vi "Periodic Tasks.vi"(8 "error in":errorcluster) -> ()   [LabVIEW 2016]
doc: "This VI runs in parallel to other tasks. It can contain as many user-defined periodic loops as you need. These can carry out PID or other sorts of timed response."
uses:
  <vilib>/Rock Robotics/SystemInterfaces/AI/FPGA_AIChannel.ctl
  <vilib>/Rock Robotics/WPI/Accelerometer/WPI_AccelerometerRange.ctl
  <vilib>/Rock Robotics/WPI/Utilities/WPI_GetSetVariantRefNum.vi
  <vilib>/Rock Robotics/WPI/Accelerometer/InternalAccelerometer/WPI_AccelerometerInternalOpen.vi
  <vilib>/Rock Robotics/WPI/Ultrasonic/WPI_SonarMB1010AnalogOpen.vi
  <vilib>/Rock Robotics/WPI/Ultrasonic/WPI_SonarMB1010AnalogRefNum Registry Set.vi
  <vilib>/Rock Robotics/WPI/Ultrasonic/WPI_SonarMB1010AnalogGetRange.vi
  <vilib>/Rock Robotics/Network Tables/NT Write Number.vi
  <vilib>/Rock Robotics/WPI/Ultrasonic/WPI_SonarMB1010AnalogClose.vi
  <vilib>/Rock Robotics/Network Tables/NT Read Boolean.vi
  <vilib>/Rock Robotics/Network Tables/NT Write Boolean.vi
panel:
  in  "Scaling Factor":dbl=0.025
  in  "Average Bits":u8=3 max=15
  out "distance":dbl(slide)=125.0 scale=0.0..250.0 scale format="%3d"
  out "error out":errorcluster
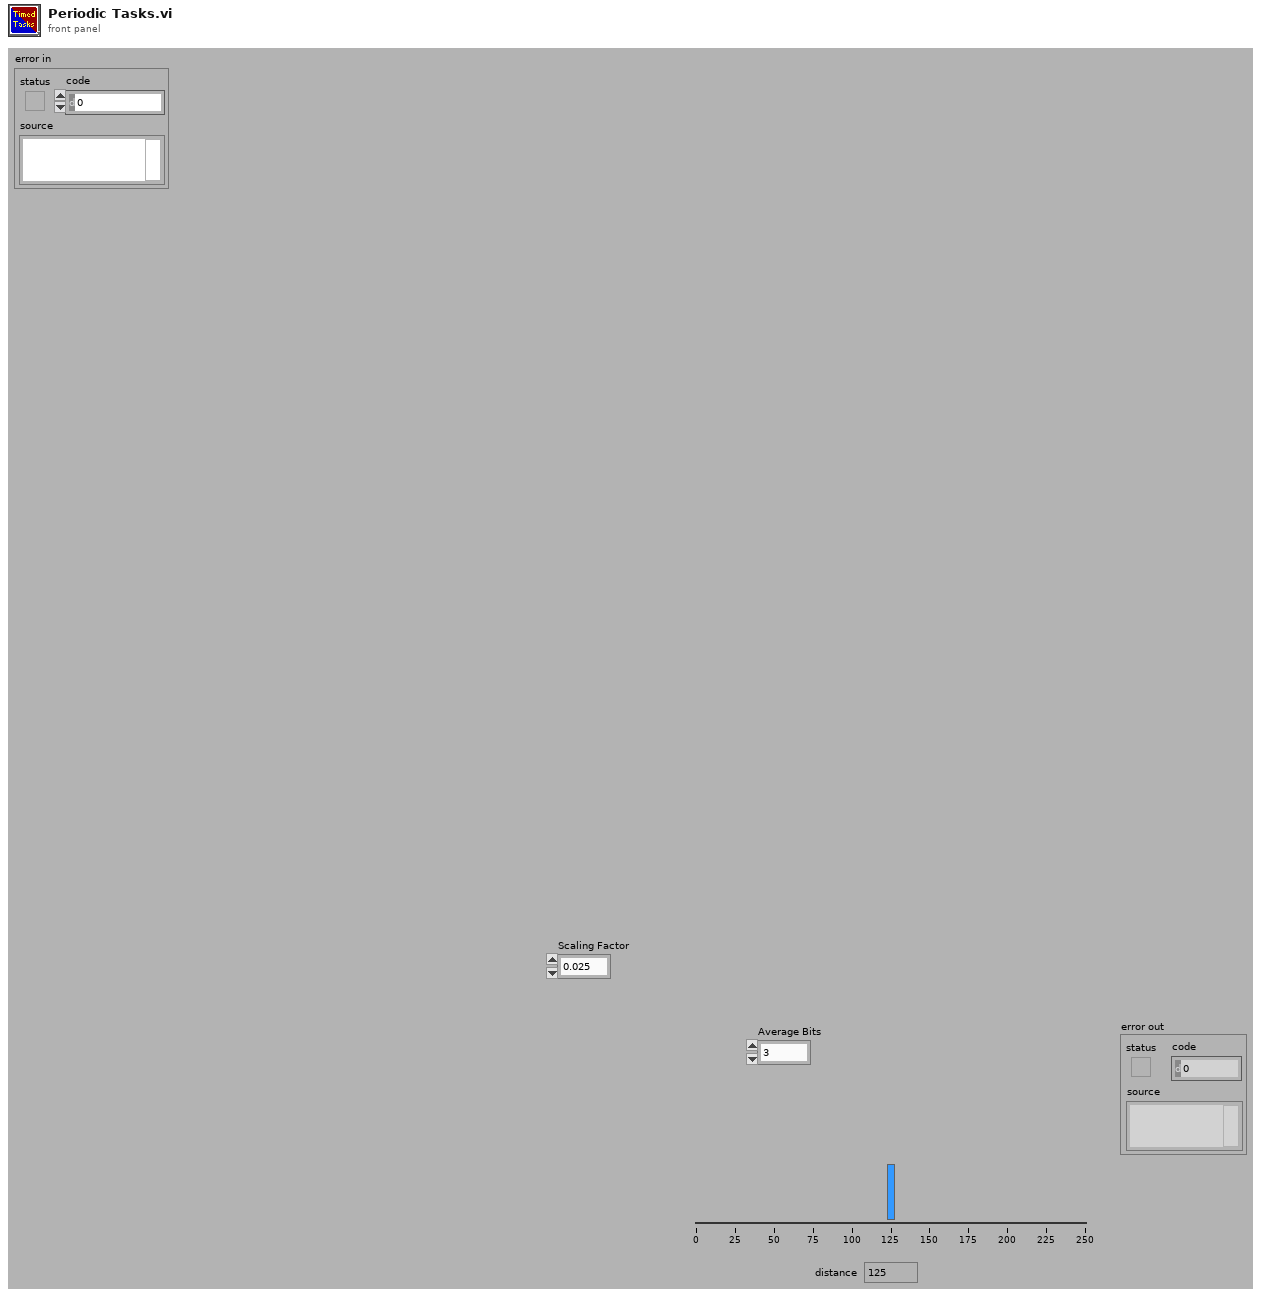
[diagram p1: front panel]
types:
  T1 = typedef "WPI_AccelerometerRange.ctl" = enum16{"+/- 2 g", "+/- 4 g", "+/- 8 g"}
  T2 = typedef "FPGA_AIChannel.ctl" = enum8{"AI 0", "AI 1", "AI 2", "AI 3", "AI MXP 0", "AI MXP 1", "AI MXP 2", "AI MXP 3", "Invalid"}
  T3 = typedef "WPI_RobotDriveDevRef.ctl" = cluster{"DevStatus":errorcluster, "Motors[]":T4[], "Square Inputs":bool, "Max Output":dbl}
  T4 = typedef "WPI_MotorControlDeviceRef.ctl" = cluster{"DeviceStatus":errorcluster, "Type":T5, "PWM":cluster{"PWM Channel":T6, "DeadBand":T7}, "CAN":cluster{"Device Number":u8, "SetOutput VI Ref":variant, "GetOutput VI Ref":variant, "Enable VI Ref":variant, "Disable VI Ref":variant, "Data":variant}, "Invert":bool}
  T5 = typedef "WPI_MotorControlType.ctl" = enum16{"PWM", "CAN"}
  T6 = typedef "FPGA_DIOPWMChannel.ctl" = enum8{"PWM 0", "PWM 1", "PWM 2", "PWM 3", "PWM 4", "PWM 5", "PWM 6", "PWM 7", "PWM 8", "PWM 9", "PWM MXP 0", "PWM MXP 1", "PWM MXP 2", "PWM MXP 3", "PWM MXP 4", "PWM MXP 5", "PWM MXP 6", "PWM MXP 7", "PWM MXP 8", "PWM MXP 9", "Invalid"}
  T7 = typedef "WPI_PWMDeadband.ctl" = cluster{"Name":string, "maxPositivePwm":i32, "minPositivePwm":i32, "centerPwm":i32, "maxNegativePwm":i32, "minNegativePwm":i32, "angularRange":u16}
  T8 = typedef "WPI_AccelerometerDevRef.ctl" = cluster{"DevStatus":errorcluster, "Scaling":T9, "Analog Channels":T10, "I2C Bus":T11, "SPI Bus":T12, "Accel Range":T13, "ADXL Axes":T14, "Handle":i32, "Device Address":u8, "Accel Type":enum16{"Analog", "ADXL345 I2C", "ADXL345 SPI", "Internal", "ADXL362 SPI"}}
  T9 = typedef "WPI_AccelerometerScaling.ctl" = cluster{"Gain (VoltsPerG)":dbl, "Center Voltage":dbl}
  T10 = typedef "WPI_AccelerometerAnalogChannels.ctl" = cluster{"X-Axis":T2, "Y-Axis":T2, "Z-Axis":T2}
  T11 = typedef "i2c_bus.ctl" = enum16{"I2C On-Board", "I2C MXP", "Invalid"}
  T12 = typedef "spi_bus.ctl" = enum16{"SPI On-Board, CS0", "SPI On-Board, CS1", "SPI On-Board, CS2", "SPI On-Board, CS3", "SPI MXP", "Invalid"}
  T13 = typedef "ADXL345 Range.ctl" = u8
  T14 = typedef "WPI_AccelerometerADXL345 Axes.ctl" = cluster{"X-Axis":bool, "Y-Axis":bool, "Z-Axis":bool}
  T15 = typedef "WPI_JoystickDevRef.ctl" = cluster{"Device":T16}
  T16 = typedef "WPI_JoystickDeviceEnum.ctl" = enum16{"USB 0", "USB 1", "USB 2", "USB 3", "USB 4", "USB 5"}
  T17 = typedef "WPI_GyroDevRef.ctl" = cluster{"DevStatus":errorcluster, "Analog Channel":T2, "Offset":dbl, "Gain (VoltsPerDegree/Second)":dbl, "Gyro Type":enum16{"Analog", "XRS450"}, "Handle":i32, "SPI Bus":T12, "Device Found":bool, "Sample Rate":dbl, "Calibrate On Open":bool}
  T18 = cluster{"JoystickDevRef":T15, "RobotDriveDevRef":T3}
  T19 = cluster{"X-Axis":dbl, "Y-Axis":dbl, "Z-Axis":dbl}
  T20 = typedef "WPI_SonarMB1010AnalogDeviceRef.ctl" = cluster{"AIDeviceRef":T21, "Scaling factor (V/in)":dbl, "Average Bits":u8}
  T21 = typedef "WPI_AnalogChannelDevRef.ctl" = cluster{"DevStatus":errorcluster, "Analog Channel":T2}
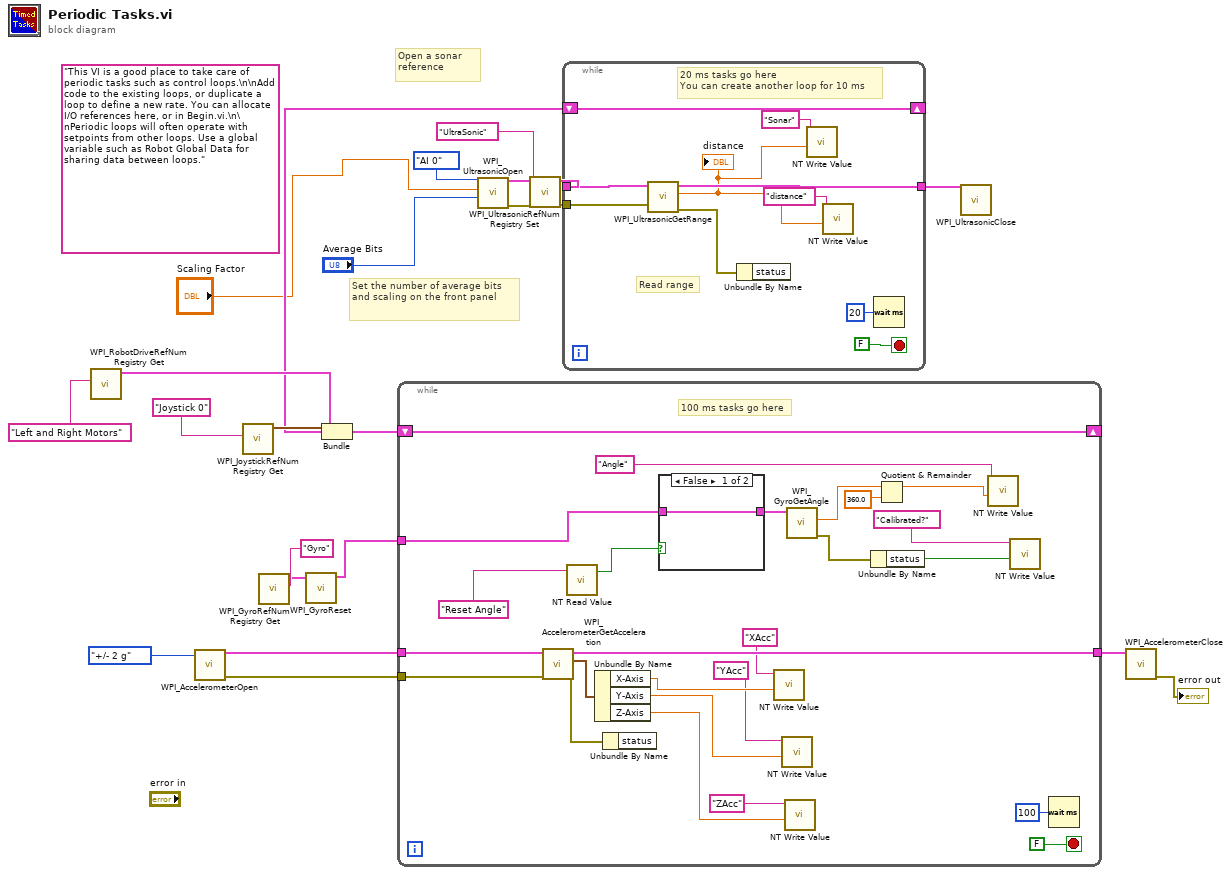
[diagram p0: block diagram]
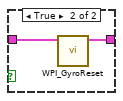
[diagram p2: hidden frame]
diagram:
  (unwired) "This VI is a good place to take care of periodic tasks such as control loops.\n\nAdd code to the existing loops, or duplicate a loop to define a new rate. You can allocate I/O references here, or in Begin.vi.\n\nPeriodic loops will often operate with setpoints from other loops. Use a global variable such as Robot Global Data for sharing data between loops."
  # "Set the number of average bits and scaling on the front panel"
  # "Open a sonar reference"
  n1 = call <vilib>:"WPI_RobotDriveRefNum Registry Get.vi"("refnum name"="Left and Right Motors") -> ("RobotDriveDevRef"=w19:T3)  [unwired: 1 in, 9 out]
  n2 = call-poly <vilib>:"WPI_AccelerometerOpen.vi"("Accel Range"=WPI_AccelerometerRange."+/- 2 g") -> ("error out"=w16:errorcluster, "AccelerometerDevRef"=w17:T8)  [unwired: 9 in]
  n3 = call <vilib>:"WPI_JoystickRefNum Registry Get.vi"("refnum name"="Joystick 0") -> ("JoystickDevRef"=w20:T15)  [unwired: 1 in, 9 out]
  n4 = call <vilib>:"WPI_GyroRefNum Registry Get.vi"("refnum name"="Gyro") -> ("GyroDevRef"=w2:T17)  [unwired: 9 in, 1 out]
  n5 = call <vilib>:"WPI_GyroReset.vi"("GyroDevRef"=w2) -> ("GyroDevRef"=w1:T17)  [unwired: 9 in, 1 out]
  n6 = Bundle("JoystickDevRef"=w20, "RobotDriveDevRef"=w19) -> (w18:T18)  [unwired: 1 out]
  n7 = while {
    shift-right: [w45] -> _
    shift-left: w18 -> [w45]
    tunnel: w17 -> [w32]
    tunnel: w16 -> [w31]
    tunnel: [w30] -> w14
    tunnel: w1 -> [w23]
    stop <- FALSE stop-if-true
    # "100 ms tasks go here"
    n8 = call <vilib>:"WPI_AccelerometerGetAcceleration.vi"("error in"=w31, "AccelerometerDevRef"=w32) -> ("error out"=w33:errorcluster, "Accelerations"=w34:T19, "AccelerometerDevRef"=w30:T8)  [unwired: 7 in]
    n9 = call-poly <vilib>:"NT Read Value.vi"("Name"="Reset Angle") -> ("Boolean"=w41:bool)  [unwired: 9 in, 1 out]
    n10 = Unbundle By Name(w34) -> ("X-Axis"=w29:dbl, "Y-Axis"=w28:dbl, "Z-Axis"=w27:dbl)
    n11 = Unbundle By Name(w33) -> ()  [unwired: 1 out]
    n12 = case shown="False" w41 {
      tunnel: [w48 w50] -> w36
      tunnel: w23 -> [w48 w49]
      frame False {
      }
      frame True {
        n13 = call <vilib>:"WPI_GyroReset.vi"("GyroDevRef"=w49) -> ("GyroDevRef"=w50:T17)  [unwired: 9 in, 1 out]
      }
    }
    n14 = call-poly <vilib>:"NT Write Value.vi"("Numeric"=w29, "Name"="XAcc") -> ()  [unwired: 9 in, 1 out]
    n15 = call-poly <vilib>:"NT Write Value.vi"("Numeric"=w28, "Name"="YAcc") -> ()  [unwired: 9 in, 1 out]
    n16 = call-poly <vilib>:"NT Write Value.vi"("Numeric"=w27, "Name"="ZAcc") -> ()  [unwired: 9 in, 1 out]
    n17 = call <vilib>:"WPI_GyroGetAngle.vi"("GyroDevRef"=w36) -> ("error out"=w38:errorcluster, "Angle"=w37:dbl)  [unwired: 6 in, 3 out]
    n18 = Unbundle By Name(w38) -> ("status"=w44:bool)
    n19 = Quotient & Remainder(x=w37, y=360.0) -> (x-y*floor(x/y)=w39:dbl)  [unwired: 1 out]
    n20 = call-poly <vilib>:"NT Write Value.vi"("Numeric"=w39, "Name"="Angle") -> ()  [unwired: 9 in, 1 out]
    n21 = call-poly <vilib>:"NT Write Value.vi"("Boolean"=w44, "Name"="Calibrated?") -> ()  [unwired: 9 in, 1 out]
    n22 = Wait (ms)(milliseconds to wait=u32 100) -> ()  [unwired: 1 out]
  }
  n23 = call-poly <vilib>:"WPI_UltrasonicOpen.vi"("Average Bits"="Average Bits", "Scaling factor (V/in)"="Scaling Factor", "Analog Channel"=FPGA_AIChannel."AI 0") -> ("error out"=w9:errorcluster, "SonarMB1010AnalogDevRef"=w7:T20)  [unwired: 7 in]
  n24 = call-poly <vilib>:"WPI_UltrasonicRefNum Registry Set.vi"("error in (no error)"=w9, "refnum name"="UltraSonic", "SonarMB1010AnalogDevRef"=w7) -> ("error out"=w5:errorcluster, "SonarMB1010AnalogDevRef"=w6:T20)  [unwired: 7 in]
  n25 = while {
    shift-right: [w58] -> _
    shift-left: w18 -> [w58]
    tunnel: [w56] -> w13
    tunnel: w6 -> [w55]
    tunnel: w5 -> [w51]
    stop <- FALSE stop-if-true
    # "Read range"
    # "20 ms tasks go here\nYou can create another loop for 10 ms"
    n26 = call-poly <vilib>:"WPI_UltrasonicGetRange.vi"("error in"=w51, "SonarMB1010AnalogDevRef"=w55) -> ("error out"=w57:errorcluster, "Distance"=w53:dbl, "SonarMB1010AnalogDevRef"=w56:T20)  [unwired: 7 in]
    "distance" <- w53
    n27 = Unbundle By Name(w57) -> ()  [unwired: 1 out]
    n28 = call-poly <vilib>:"NT Write Value.vi"("Numeric"=w53, "Name"="Sonar") -> ()  [unwired: 9 in, 1 out]
    n29 = call-poly <vilib>:"NT Write Value.vi"("Numeric"=w53, "Name"="distance") -> ()  [unwired: 9 in, 1 out]
    n30 = Wait (ms)(milliseconds to wait=u32 20) -> ()  [unwired: 1 out]
  }
  n31 = call-poly <vilib>:"WPI_UltrasonicClose.vi"("SonarMB1010AnalogDevRef"=w13) -> ()  [unwired: 10 in, 1 out]
  n32 = call <vilib>:"WPI_AccelerometerClose.vi"("AccelerometerDevRef"=w14) -> ("error out"=→"error out":errorcluster)  [unwired: 10 in]
